vi "User Interface.vi"(8 "error in (no error)":errorcluster, 11 "User Interface in":refnum<class "User Interface.lvclass">) -> (0 "error out":errorcluster, 3 "User Interface out":refnum<class "User Interface.lvclass">)   [LabVIEW 2017, in "GE Reflective Memory.lvlib" / "Thread User Interface.lvclass"]
uses:
  Thread User Interface.lvclass
  DSF Core.lvlibp/Classes/User Interface/User Interface.lvclass
  Configurations/Thread/Thread Configuration.lvclass
  Configurations/Thread/Thread Configuration.lvclass/Thread Configuration.ctl
  C:/Git/DSF/Components/DSF Core.lvlibp/Classes/Configuration/Configuration.lvclass
panel:
  in  "DMA Wait Mode":enum16{"Polling", "Interrupt"}(ring)
  in  "VISA Resource":string
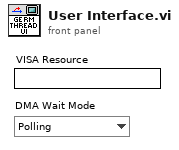
[diagram p1: front panel]
types:
  T1 = typedef "GE 5565PIORC.lvclass/GE 5565PIORC.Typedef.DMA Wait Mode.ctl" = enum16{"Polling", "Interrupt"}
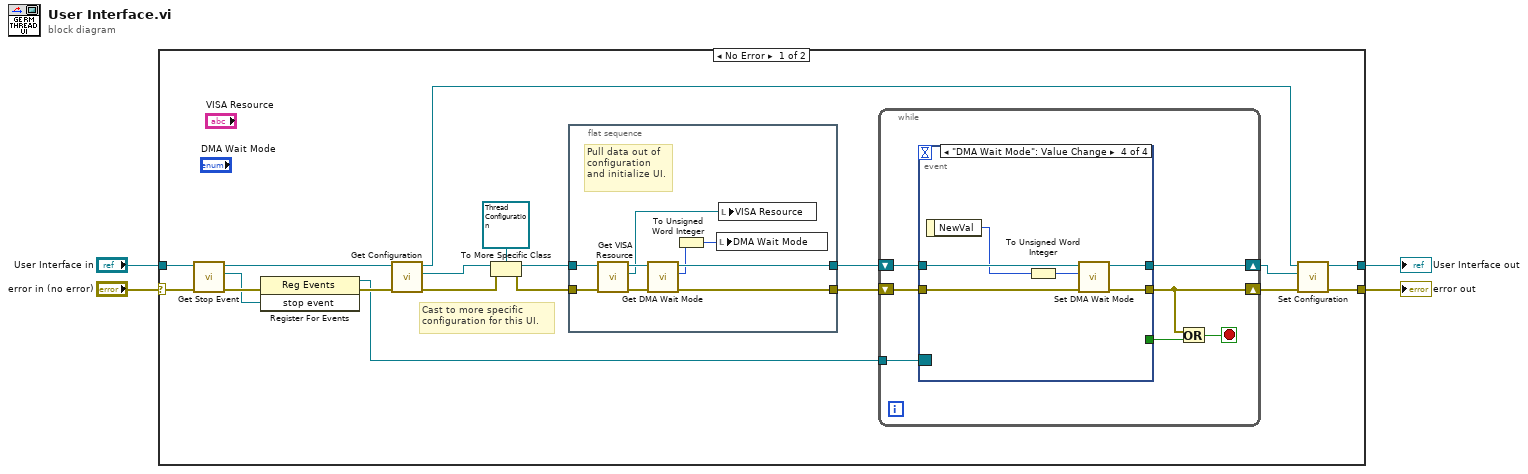
[diagram p0: block diagram]
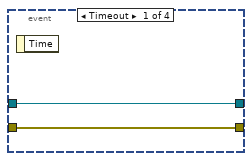
[diagram p2: hidden frame]
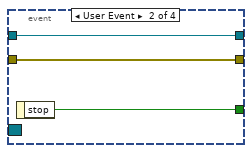
[diagram p3: hidden frame]
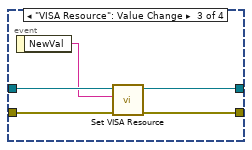
[diagram p4: hidden frame]
diagram:
  n1 = case shown="No Error" "error in (no error)" {
    selector: "error in (no error)" -> [w19 w57]
    tunnel: [w7 w57] -> w4
    tunnel: "User Interface in" -> [w18 w56]
    tunnel: [w6 w56] -> w1
    frame No Error {
      # "Cast to more specific configuration for this UI."
      n2 = call "Get Stop Event.vi"("error in (no error)"=w19, "User Interface in"=w18) -> ("error out"=w17:errorcluster, "stop event"=w16:refnum<user-event>, "User Interface out"=w15:refnum<class "User Interface.lvclass">)  [unwired: 7 in]
      n3 = register-events(error in=w17, w16) -> (reference out=w13:refnum<event-registration>, error out=w14:errorcluster)  [unwired: 1 in]
      n4 = call "Get Configuration.vi"("error in (no error)"=w14, "User Interface in"=w15) -> ("error out"=w12:errorcluster, "configuration"=w10:refnum<class "Configuration.lvclass">, "User Interface out"=w5:refnum<class "User Interface.lvclass">)  [unwired: 7 in]
      n5 = To More Specific Class(target class=refnum<class "Thread Configuration.lvclass"> refnum ("Configuration out"), reference=w10, error in=w12) -> (specific class reference=w23:refnum<class "Thread Configuration.lvclass">, error out=w20:errorcluster)
      n6 = flat-sequence {
        tunnel: [w27] -> w21
        tunnel: w20 -> [w32]
        tunnel: w23 -> [w31]
        tunnel: [w28] -> w22
        frame #0 {
          # "Pull data out of configuration and initialize UI."
          n7 = call "Get VISA Resource.vi"("error in (no error)"=w32, "Thread Configuration in"=w31) -> ("error out"=w29:errorcluster, "VISA Resource"=w26:refnum<visa-resource-name>, "Thread Configuration out"=w30:refnum<class "Thread Configuration.lvclass">)  [unwired: 7 in]
          n8 = call "Get DMA Wait Mode.vi"("error in (no error)"=w29, "Thread Configuration in"=w30) -> ("error out"=w27:errorcluster, "wait mode"=w25:T1, "Thread Configuration out"=w28:refnum<class "Thread Configuration.lvclass">)  [unwired: 7 in]
          n9 = To Unsigned Word Integer(number=w25) -> (unsigned 16bit integer=w24:u16)
          n10 = local write "DMA Wait Mode"(w24) -> ()
          n11 = local write "VISA Resource"(w26) -> ()
        }
      }
      n12 = while {
        tunnel: w13 -> [w39]
        shift-right: [w37] -> w8
        shift-left: w21 -> [w38]
        shift-right: [w33] -> w9
        shift-left: w22 -> [w34]
        stop <- w36 stop-if-true
        n13 = event shown="[3] \"DMA Wait Mode\": Value Change" {
          selector: w39 -> [_ _ _ _]
          dyn-events: _ -> [_ _ _ _]
          timeout: _ -> [_ _ _ _]
          tunnel: [_ w42 _ _] -> w35
          tunnel: w38 -> [w41 w44 w49 w52]
          tunnel: [w41 w44 w46 w53] -> w37
          tunnel: w34 -> [w40 w43 w48 w55]
          tunnel: [w40 w43 w45 w54] -> w33
          event Timeout {
            n14 = event-data() -> ()  [unwired: 1 in, 1 out]
          }
          event User Event {
            n15 = event-data() -> ("stop"=w42:bool)  [unwired: 1 in]
          }
          event "VISA Resource": Value Change {
            n16 = event-data() -> ("NewVal"=w47:string)  [unwired: 1 in]
            n17 = call "Set VISA Resource.vi"("error in (no error)"=w49, "VISA Resource"=w47, "Thread Configuration in"=w48) -> ("error out"=w46:errorcluster, "Thread Configuration out"=w45:refnum<class "Thread Configuration.lvclass">)  [unwired: 7 in]
          }
          event "DMA Wait Mode": Value Change {
            n18 = event-data() -> ("NewVal"=w51:enum16{"Polling", "Interrupt"})  [unwired: 1 in]
            n19 = To Unsigned Word Integer(number=w51) -> (unsigned 16bit integer=w50:u16)
            n20 = call "Set DMA Wait Mode.vi"("error in (no error)"=w52, "wait mode"=w50, "Thread Configuration in"=w55) -> ("error out"=w53:errorcluster, "Thread Configuration out"=w54:refnum<class "Thread Configuration.lvclass">)  [unwired: 7 in]
          }
        }
        n21 = Or(x=w37, y=w35) -> (x .or. y?=w36:bool)
      }
      n22 = call "Set Configuration.vi"("error in (no error)"=w8, "configuration"=w9, "User Interface in"=w5) -> ("error out"=w7:errorcluster, "User Interface out"=w6:refnum<class "User Interface.lvclass">)  [unwired: 7 in]
    }
    frame Error {
    }
  }
  "error out" <- w4
  "User Interface out" <- w1
